vi "InitializeAIchannel.vi.vi"(8 "error in (no error)":errorcluster, 11 "config in":T1 {"HighPassFilterState"."Filter State" format="%.2f"; "HighPassFilterState"."IIR Filter Cluster"."Forward Coefficients" format="%.2f"; "HighPassFilterState"."IIR Filter Cluster"."Reverse Coefficients" format="%.2f"; "FixedSizeX32"."InputConfig" items=["AC Coupled", "DC Coupled", "IEPE AC Coupled"]}) -> (0 "error out":errorcluster, 2 "cDAQ with TSN AI Channel(s)":tag, 3 "config out":T1 {"HighPassFilterState"."Filter State" format="%.2f"; "HighPassFilterState"."IIR Filter Cluster"."Forward Coefficients" format="%.2f"; "HighPassFilterState"."IIR Filter Cluster"."Reverse Coefficients" format="%.2f"; "FixedSizeX32"."InputConfig" items=["AC Coupled", "DC Coupled", "IEPE AC Coupled"]})   [LabVIEW 2017, in "TSNcDAQ_AI.lvlib"]
uses:
  <vilib>/addons/InsightCM/Devices/Shared/Cms/DAQmx/TSNcDAQ_AI.lvlib
  <vilib>/addons/InsightCM/Devices/Shared/Cms/CmsAcquisition/controls/Configuration.ctl
  <vilib>/addons/InsightCM/Devices/Shared/Cms/CmsAcquisition/controls/TachometerConfig.ctl
  <vilib>/addons/InsightCM/Devices/Shared/Cms/CmsAcquisition/controls/FixedSizeArrays.ctl
  <vilib>/LabVIEW Targets/FPGA/cRIO/shared/nicrio_ModuleControls/nicrio_cRIO-9232_ConfigModeRing.ctl
  <vilib>/addons/InsightCM/Devices/Shared/Cms/cRIOWfmAcq/subVIs/RIO Wfm Cust Ctrls/rwfm_SamplingInfo.ctl
  <vilib>/addons/InsightCM/Devices/Shared/Cms/CmsAcquisition/controls/Group.ctl
  <vilib>/addons/InsightCM/Devices/Shared/Cms/CmsAcquisition/controls/Channel.ctl
  <vilib>/addons/InsightCM/Utilities/Analysis/Vibration/controls/HighPassFilterState.ctl
  <vilib>/addons/InsightCM/Devices/Shared/Cms/CmsAcquisition/controls/BurstMode.ctl
  <vilib>/addons/cRIODetectHW/cRIODetectHW.lvlib
  <vilib>/addons/SystemInfoProcess/SystemInfoProcess.lvlib
  <vilib>/addons/InsightCM/Devices/Shared/Cms/CmsAcquisition/CmsAcquisition.lvlib
  <vilib>/addons/InsightCM/Devices/Shared/Cms/cRIOWfmAcq/cRIOWfmLib.lvlib
  <vilib>/addons/InsightCM/Utilities/Analysis/Vibration/VibrationAnalysisFunctions.lvlib
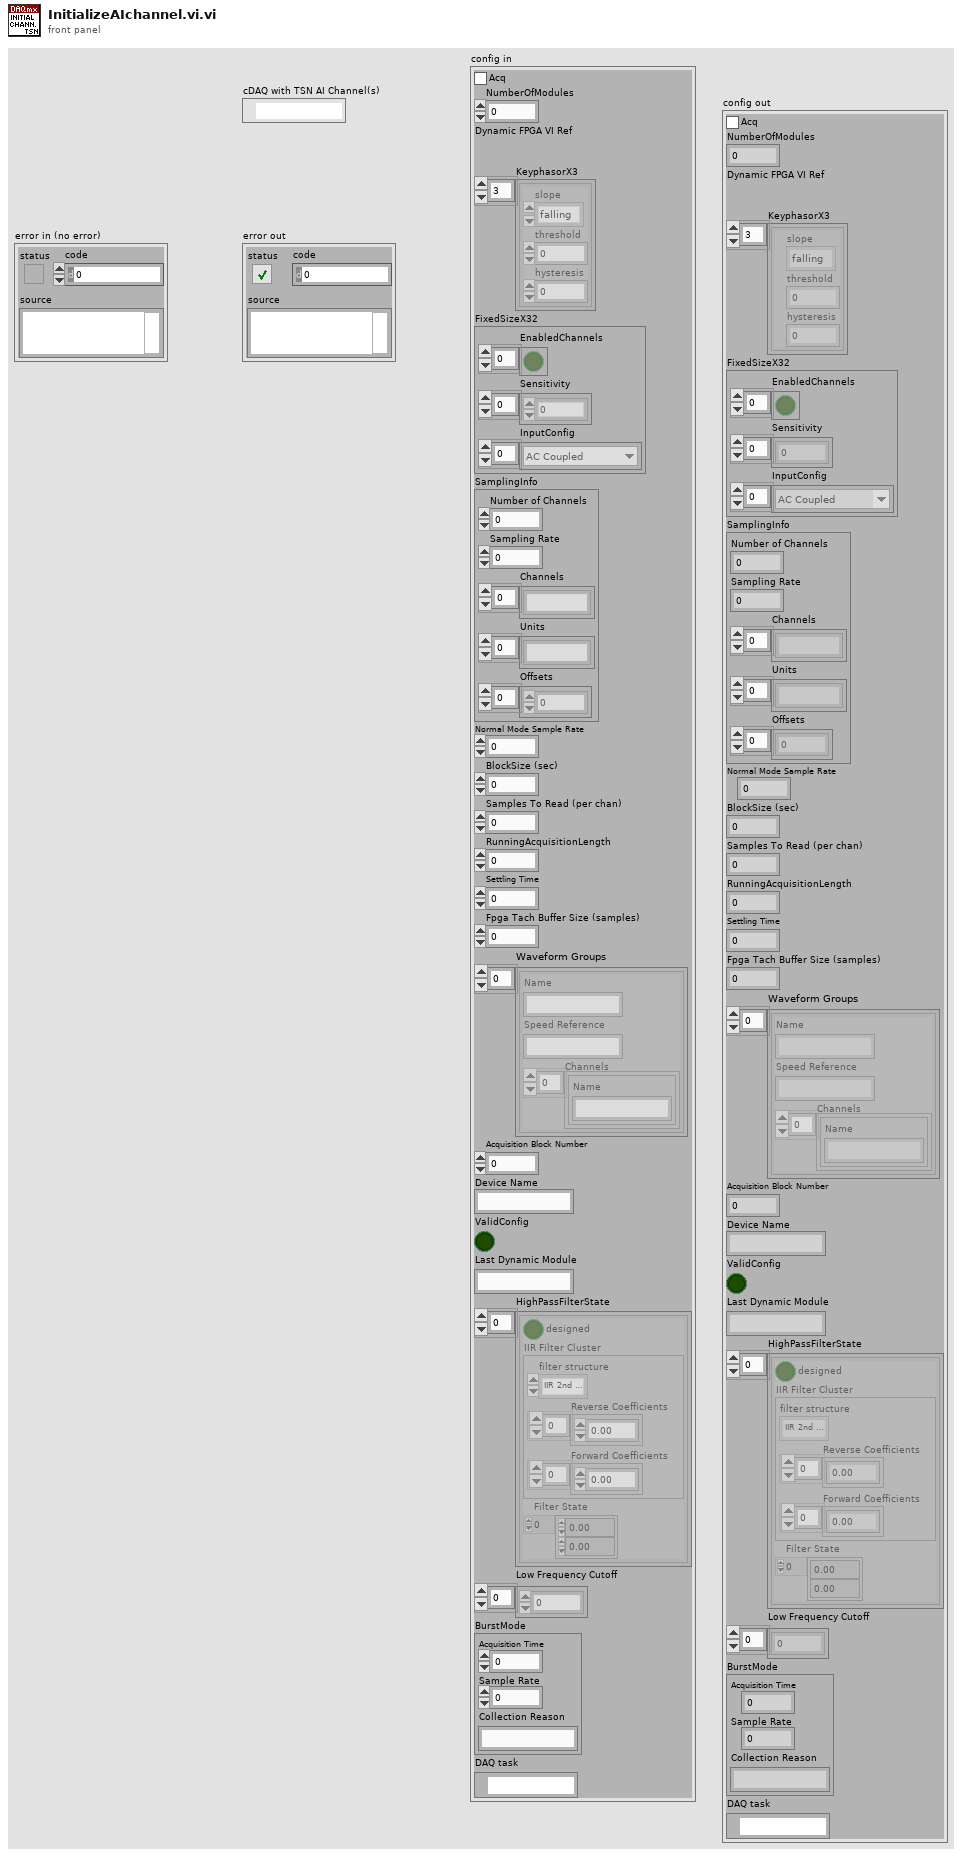
[diagram p1: front panel]
types:
  T1 = typedef "CmsAcquisition.lvlib/Configuration.ctl" = cluster{"Acq":bool, "NumberOfModules":i16, "Dynamic FPGA VI Ref":refnum<k20>, "KeyphasorX3":T2[], "FixedSizeX32":T3, "SamplingInfo":T5, "Normal Mode Sample Rate":dbl, "BlockSize (sec)":dbl, "Samples To Read (per chan)":i32, "RunningAcquisitionLength":dbl, "Settling Time":dbl, "Fpga Tach Buffer Size (samples)":i32, "Waveform Groups":T6[], "Acquisition Block Number":i32, "Device Name":string, "ValidConfig":bool, "Last Dynamic Module":string, "HighPassFilterState":T8[], "Low Frequency Cutoff":dbl[], "BurstMode":T9, "DAQ task":refnum<k21>}
  T2 = typedef "CmsAcquisition.lvlib/TachometerConfig.ctl" = cluster{"slope":enum16{"falling", "rising"}, "threshold":dbl, "hysteresis":dbl}
  T3 = typedef "CmsAcquisition.lvlib/FixedSizeArrays.ctl" = cluster{"EnabledChannels":bool[], "Sensitivity":dbl[], "InputConfig":T4[]}
  T4 = typedef "nicrio_cRIO-9232_ConfigModeRing.ctl" = u8
  T5 = typedef "cRIOWfmLib.lvlib/rwfm_SamplingInfo.ctl" = cluster{"Number of Channels":i32, "Sampling Rate":dbl, "Channels":string[], "Units":string[], "Offsets":sgl[]}
  T6 = typedef "CmsAcquisition.lvlib/Group.ctl" = cluster{"Name":string, "Speed Reference":string, "Channels":T7[]}
  T7 = typedef "CmsAcquisition.lvlib/Channel.ctl" = cluster{"Name":string}
  T8 = typedef "VibrationAnalysisFunctions.lvlib/HighPassFilterState.ctl" = cluster{"designed":bool, "IIR Filter Cluster":cluster{"filter structure":enum32{"IIR 2nd Order", "IIR 4th Order"}, "Reverse Coefficients":dbl[], "Forward Coefficients":dbl[]}, "Filter State":dbl[]}
  T9 = typedef "CmsAcquisition.lvlib/BurstMode.ctl" = cluster{"Acquisition Time":dbl, "Sample Rate":dbl, "Collection Reason":string}
  T10 = typedef "cRIODetectHW.lvlib/SystemHW.ctl" = cluster{"controller":T11, "chassis":T11, "modules":T11[]}
  T11 = typedef "cRIODetectHW.lvlib/cRIO Product Info.ctl" = cluster{"vendorName":string, "productName":string, "serialNumber":string}
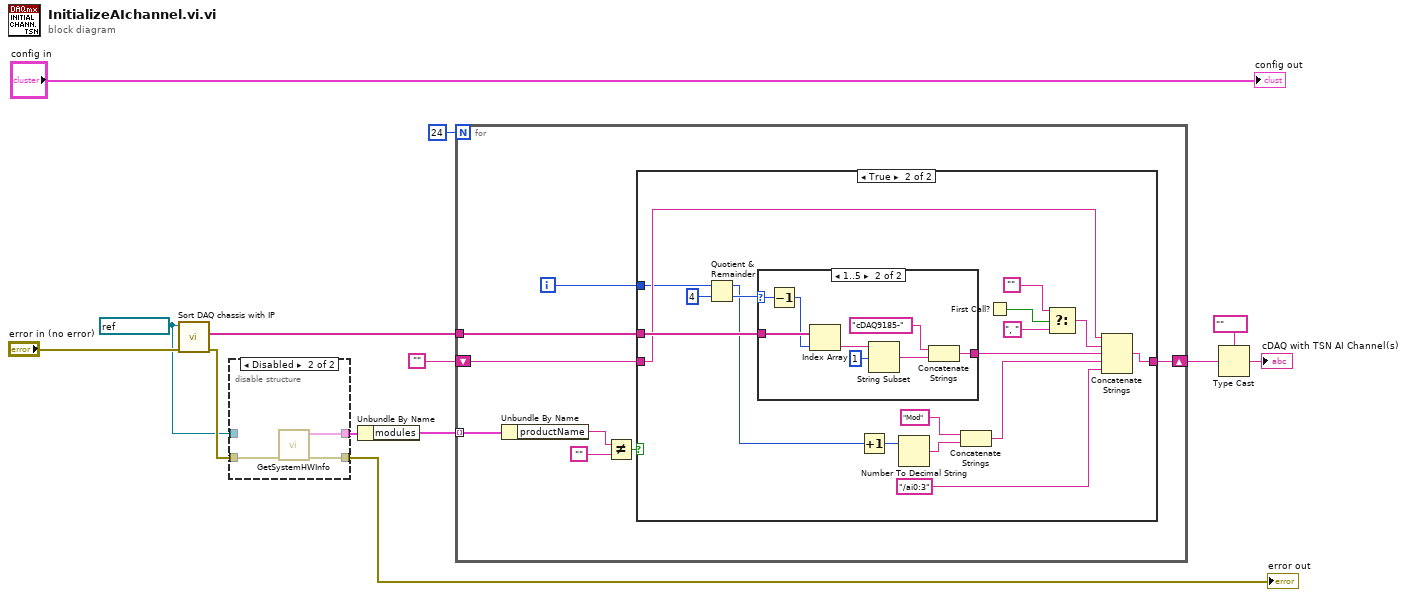
[diagram p0: block diagram]
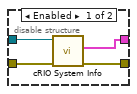
[diagram p2: hidden frame]
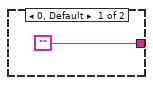
[diagram p4: hidden frame]
diagram:
  w1 = refnum<k21> "localhost" ("Target (localhost)")
  n1 = call <vilib>:"Sort DAQ chassis with IP.vi"("error in (no error)"="error in (no error)", "Target (localhost)"=w1) -> ("error out"=w8:errorcluster, "SN Number"=w11:string[])  [unwired: 8 in]
  n2 = disable-structure shown="Disabled" {
    disable-tunnel: [w17 w19] -> w9
    disable-tunnel: w8 -> [w16 w20]
    disable-tunnel: [w15 w18] -> w6
    disable-tunnel: w1 -> [w14 _]
    frame Enabled {
      n3 = call <vilib>:"cRIO System Info.vi"("error in (no error)"=w16, "session in"=w14) -> ("error out"=w15:errorcluster, "system info"=w17:T10)  [unwired: 8 in]
    }
    frame Disabled {
      n4 = call <vilib>:"GetSystemHWInfo.vi"("error in (no error)"=w20) -> ("error out"=w18:errorcluster, "system info"=w19:T10)  [unwired: 8 in, 1 out]
    }
  }
  "error out" <- w6
  n5 = Unbundle By Name(w9) -> ("modules"=w13:T11[])
  n6 = for {
    N: 24 -> [_]
    tunnel: w13 -> [w28] mode=indexing
    tunnel: w11 -> [w24]
    shift-right: [w21] -> w5
    shift-left: "" -> [w22]
    i -> [w25]
    n7 = Unbundle By Name(w28) -> ("productName"=w27:string)
    n8 = Not Equal?(x=w27, y="") -> (x != y?=w23:bool)
    n9 = case shown="True" w23 {
      tunnel: w25 -> [_ w30]
      tunnel: w24 -> [_ w44]
      tunnel: [w29 w36] -> w21
      tunnel: w22 -> [w29 w35]
      frame False {
      }
      frame True {
        n10 = Quotient & Remainder(x=w30, y=4) -> (x-y*floor(x/y)=w43:i32, floor(x/y)=w45:i32)
        n11 = case shown="1..5" w45 {
          selector: w45 -> [_ w54]
          tunnel: w44 -> [_ w55]
          tunnel: ["" w48] -> w39
          frame 0, Default {
          }
          frame 1..5 {
            n12 = Decrement(x=w54) -> (x-1=w53:i32)
            n13 = Index Array(array=w55, index=w53) -> (element=w52:string)
            n14 = String Subset(string=w52, offset (0)=1) -> (substring=w49:string)  [unwired: 1 in]
            n15 = Concatenate Strings("cDAQ9185-", w49) -> (w48:string)
          }
        }
        n16 = Increment(x=w43) -> (x+1=w42:i32)
        n17 = Number To Decimal String(number=w42) -> (decimal integer string=w40:string)  [unwired: 1 in]
        n18 = Concatenate Strings("Mod", w40) -> (w38:string)
        n19 = First Call?() -> (First Call?: T/F=w34:bool)
        n20 = Select(t="", s=w34, f=", " ("string")) -> (s? t:f=w32:string)
        n21 = Concatenate Strings(w35, w32, w39, w38, "/ai0:3") -> (w36:string)
      }
    }
  }
  n22 = Type Cast(type=tag "" ("AI Channel(s)"), x=w5) -> (*(type *) &x=→"cDAQ with TSN AI Channel(s)":tag)
  "config out" <- "config in"
